vi "纳清pH_所有参数读取.vi"(8 "error in (no error)":errorcluster caption="错误输入（无错误）", 11 "MB session in":refnum<class "MB_Master.lvclass">) -> (0 "error out":errorcluster caption="错误输出", 2 "输出值":T1 {"波特率" items=["4800", "9600", "19200", "38400", "57600", "115200"]}, 3 "MB session out":refnum<class "MB_Master.lvclass">)   [LabVIEW 2016, in "斯坦道多参数.lvlib"]
uses:
  <vilib>/Plasmionique/MB Master/MB_Master/MB_Master.lvclass
  <vilib>/Plasmionique/MB Master/MB Master.lvlib
  <vilib>/ptbypt/NI_PtbyPt.lvlib
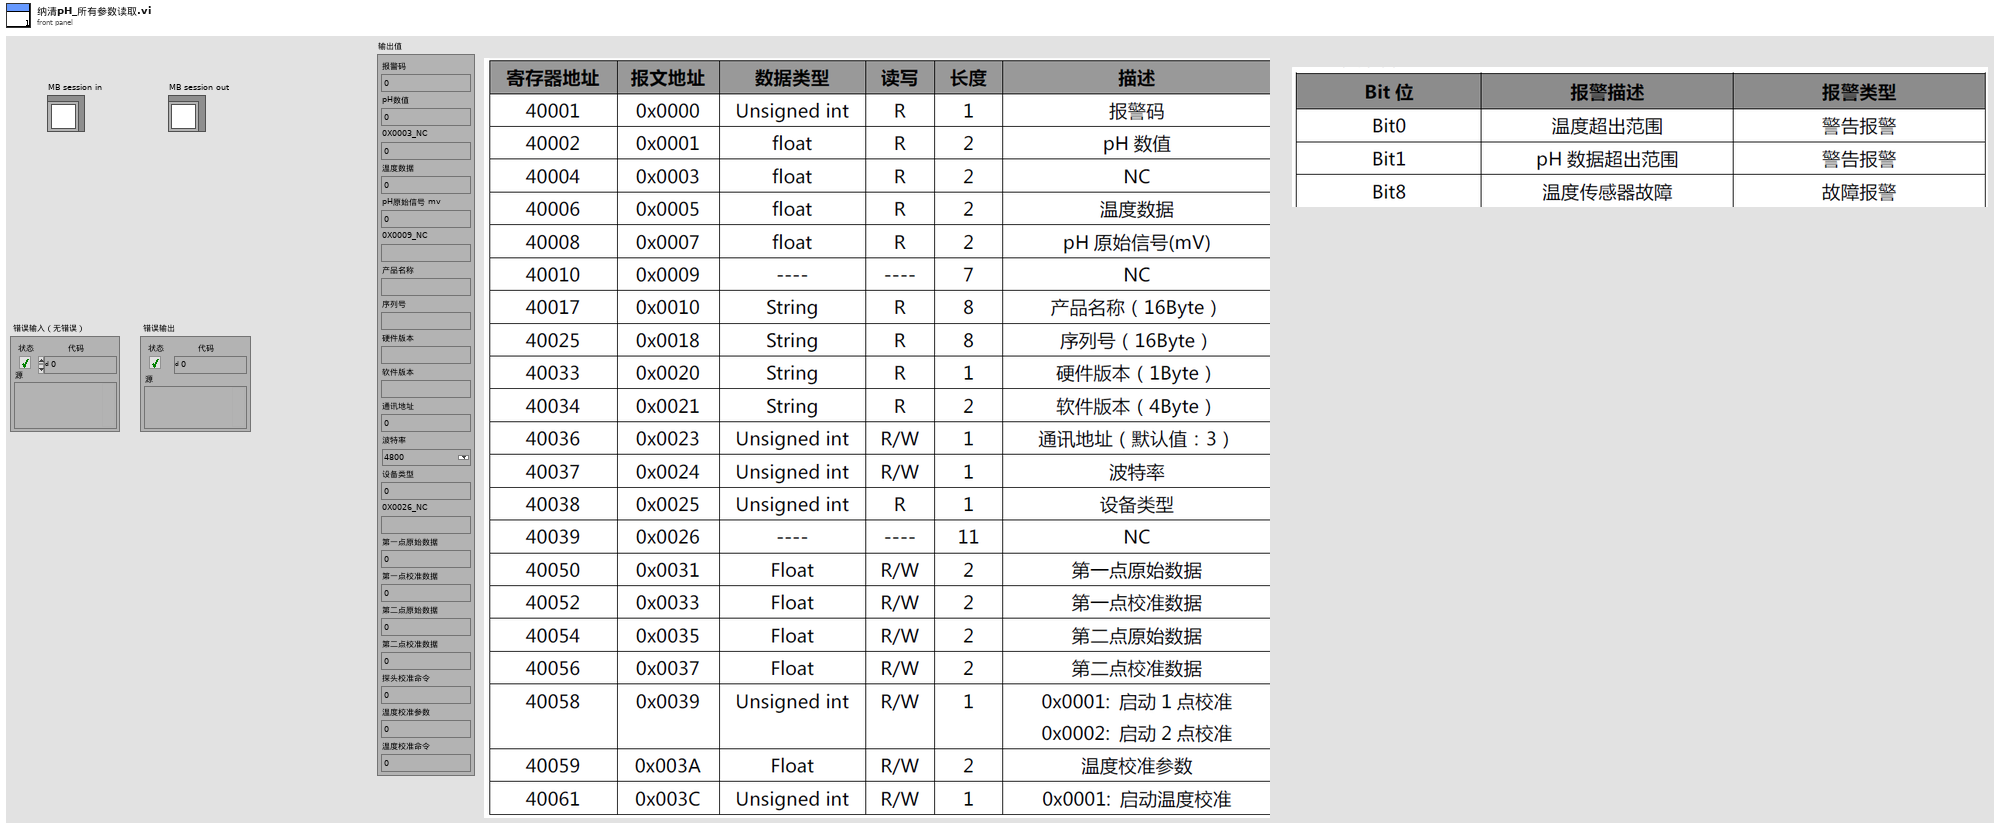
[diagram p1: front panel]
types:
  T1 = cluster{"报警码":u16, "pH数值":sgl, "0X0003_NC":sgl, "温度数据":sgl, "pH原始信号 mv":sgl, "0X0009_NC":string, "产品名称":string, "序列号":string, "硬件版本":string, "软件版本":string, "通讯地址":u16, "波特率":u16, "设备类型":u16, "0X0026_NC":string, "第一点原始数据":sgl, "第一点校准数据":sgl, "第二点原始数据":sgl, "第二点校准数据":sgl, "探头校准命令":u16, "温度校准参数":sgl, "温度校准命令":u16}
  T2 = cluster{u16, "Filtered x":dbl, "数值":sgl, "数值":sgl, "数值":sgl, "类型":string, "类型":string, "类型":string, "类型":string, "类型":string, u16, u16, u16, "类型":string, "数值":sgl, "数值":sgl, "数值":sgl, "数值":sgl, u16, "数值":sgl, u16}
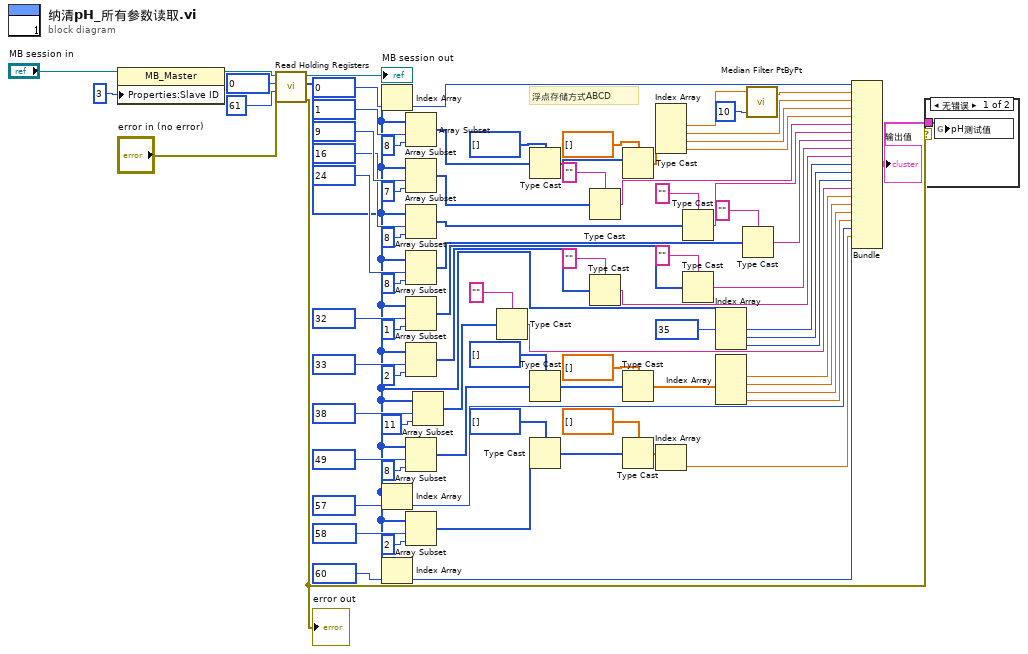
[diagram p0: block diagram]
diagram:
  # "浮点存储方式ABCD"
  n1 = property class="MB_Master"(reference="MB session in", "Properties:Slave ID"=u8 3 ("Slave ID")) -> (reference out=w72:refnum<class "MB_Master.lvclass">)  [unwired: 1 in, 1 out]
  n2 = call <vilib>:"Read Holding Registers.vi"("error in (no error)"="error in (no error)", "quantity"=u16 61, "starting address"=u16 0, "MB session in"=w72) -> ("error out"=w13:errorcluster, "Registers"=w15:u16[], "MB session out"=→"MB session out":refnum<class "MB_Master.lvclass">)  [unwired: 5 in]
  "error out" <- w13
  n3 = Index Array(array=w15, index=u16 0 ("starting address")) -> (element=w80:u16)
  n4 = Index Array(array=w15, index=u16 57 ("starting address")) -> (element=w18:u16)
  n5 = Index Array(array=w15, index=u16 60 ("starting address")) -> (element=w14:u16)
  n6 = Array Subset(array=w15, index=u16 1 ("starting address"), length=8 ("长度")) -> (w76:u16[])
  n7 = Array Subset(array=w15, index=u16 9 ("starting address"), length=7 ("长度")) -> (w66:u16[])
  n8 = Array Subset(array=w15, index=u16 16 ("starting address"), length=8 ("长度")) -> (w62:u16[])
  n9 = Array Subset(array=w15, index=u16 24 ("starting address"), length=8 ("长度")) -> (w56:u16[])
  n10 = Array Subset(array=w15, index=u16 32 ("starting address"), length=1 ("长度")) -> (w52:u16[])
  n11 = Array Subset(array=w15, index=u16 33 ("starting address"), length=2 ("长度")) -> (w46:u16[])
  n12 = Array Subset(array=w15, index=u16 49 ("starting address"), length=8 ("长度")) -> (w33:u16[])
  n13 = Array Subset(array=w15, index=u16 58 ("starting address"), length=2 ("长度")) -> (w21:u16[])
  n14 = Array Subset(array=w15, index=u16 38 ("starting address"), length=11 ("长度")) -> (w36:u16[])
  n15 = Type Cast(type="" ("类型"), x=w36) -> (*(type *) &x=w35:string)
  n16 = Type Cast(type=u32[] [] ("数组 2"), x=w76) -> (*(type *) &x=w12:u32[])
  n17 = Type Cast(type=u32[] [] ("数组 2"), x=w33) -> (*(type *) &x=w31:u32[])
  n18 = Type Cast(type=u32[] [] ("数组 2"), x=w21) -> (*(type *) &x=w23:u32[])
  n19 = Type Cast(type="" ("类型"), x=w66) -> (*(type *) &x=w64:string)
  n20 = Type Cast(type="" ("类型"), x=w46) -> (*(type *) &x=w44:string)
  n21 = Type Cast(type=sgl[] [] ("数组 2"), x=w12) -> (*(type *) &x=w75:sgl[])
  n22 = Type Cast(type=sgl[] [] ("数组 2"), x=w31) -> (*(type *) &x=w28:sgl[])
  n23 = Type Cast(type=sgl[] [] ("数组 2"), x=w23) -> (*(type *) &x=w26:sgl[])
  n24 = Index Array(array=w75) -> (element #1=w2:sgl, element #2=w70:sgl, element #3=w9:sgl, element #4=w8:sgl)  [unwired: 4 in]
  n25 = Index Array(array=w26) -> (element=w17:sgl)  [unwired: 1 in]
  n26 = Type Cast(type="" ("类型"), x=w62) -> (*(type *) &x=w59:string)
  n27 = Type Cast(type="" ("类型"), x=w52) -> (*(type *) &x=w49:string)
  n28 = Index Array(array=w15, index #1=u16 35 ("starting address")) -> (element #1=w42:u16, element #2=w41:u16, element #3=w40:u16)  [unwired: 2 in]
  n29 = Index Array(array=w28) -> (element #1=w27:sgl, element #2=w7:sgl, element #3=w6:sgl, element #4=w5:sgl)  [unwired: 4 in]
  n30 = Type Cast(type="" ("类型"), x=w56) -> (*(type *) &x=w54:string)
  n31 = call <vilib>:"Median Filter PtByPt.vi"("rank"=10, "x"=w2) -> ("Filtered x"=w1:dbl)  [unwired: 2 in, 1 out]
  n32 = Bundle(w80, "Filtered x"=w1, "数值"=w70, "数值"=w9, "数值"=w8, "类型"=w64, "类型"=w59, "类型"=w54, "类型"=w49, "类型"=w44, w42, w41, w40, "类型"=w35, "数值"=w27, "数值"=w7, "数值"=w6, "数值"=w5, w18, "数值"=w17, w14) -> (w4:T2)  [unwired: 1 in]
  "输出值" <- w4
  n33 = case shown="无错误" w13 {
    tunnel: w4 -> [w83 _]
    frame No Error {
      n34 = global write "纳清过程全局变量.vi" "pH测试值"(w83) -> ()
    }
    frame Error {
    }
  }
